vi "DrivePID.vi"(0 "Ldrive Encoder":dbl, 5 "Rdrive Encoder":dbl, 7 "Compensate":bool, 9 "SetpointLeft":dbl format="%.2f", 11 "SetpointRight":dbl format="%.2f") -> (6 "Left Out":dbl, 8 "Right Out":dbl, 15 "Done":bool)   [LabVIEW 2015]
uses:
  <vilib>/addons/control/pid/pid.llb/PID (DBL).vi
  <vilib>/addons/control/pid/NI_PID_pid.lvlib
panel:
  in  "Max Speed":dbl=0.5
  in  "RightDriveRefNum":string="My Encoder RefNum"
  in  "LeftDriveRefNum":string="My Encoder RefNum"
  in  "PID gains for motor gain":T1={"proportional gain (Kc)"=1.0, "integral time (Ti, min)"=0.01, "derivative time (Td, min)"=0.0} {"derivative time (Td, min)" format="%.3f"; "integral time (Ti, min)" format="%.3f"; "proportional gain (Kc)" format="%.3f"}
  in  "PID gains Right":T1={"proportional gain (Kc)"=0.6, "integral time (Ti, min)"=0.0055, "derivative time (Td, min)"=0.001} {"derivative time (Td, min)" format="%.3f"; "integral time (Ti, min)" format="%.7f"; "proportional gain (Kc)" format="%.3f"}
  out "Right Chart":dbl(graph)
  out "Left Chart":dbl(graph)
  in  "PID gains Left":T1={"proportional gain (Kc)"=0.6, "integral time (Ti, min)"=0.0055, "derivative time (Td, min)"=0.001} {"derivative time (Td, min)" format="%.3f"; "integral time (Ti, min)" format="%.7f"; "proportional gain (Kc)" format="%.3f"}
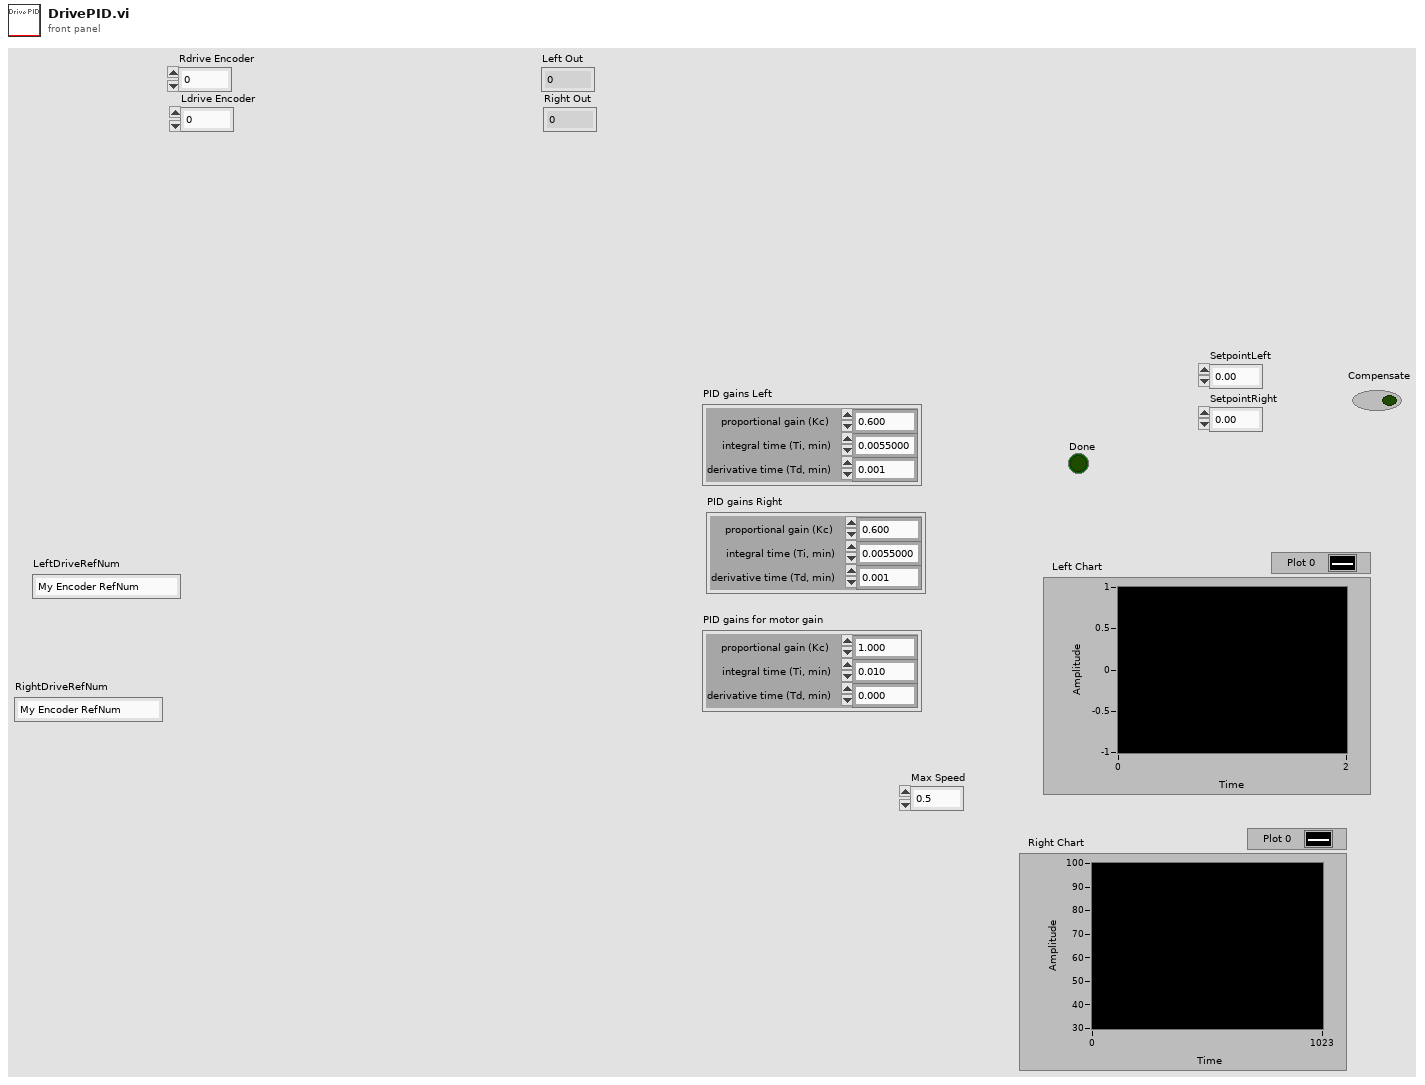
[diagram p1: front panel]
types:
  T1 = cluster{"proportional gain (Kc)":dbl, "integral time (Ti, min)":dbl, "derivative time (Td, min)":dbl}
  T2 = typedef "WPI_EncoderDevRef.ctl" = cluster{"DevStatus":errorcluster, "EncoderIndex":T3, "CounterIndex":T4, "DistancePerCount":dbl, "Decoding Type":T5}
  T3 = typedef "FPGA_EncoderIdx.ctl" = enum8{"Enc 0", "Enc 1", "Enc 2", "Enc 3", "Enc 4", "Enc 5", "Enc 6", "Enc 7", "Invalid"}
  T4 = typedef "FPGA_CounterCtrSystemIndex.ctl" = enum8{"Ctr 0", "Ctr 1", "Ctr 2", "Ctr 3", "Ctr 4", "Ctr 5", "Ctr 6", "Ctr 7", "Invalid"}
  T5 = typedef "WPI_EncoderType.ctl" = enum16{"1x", "2x", "4x"}
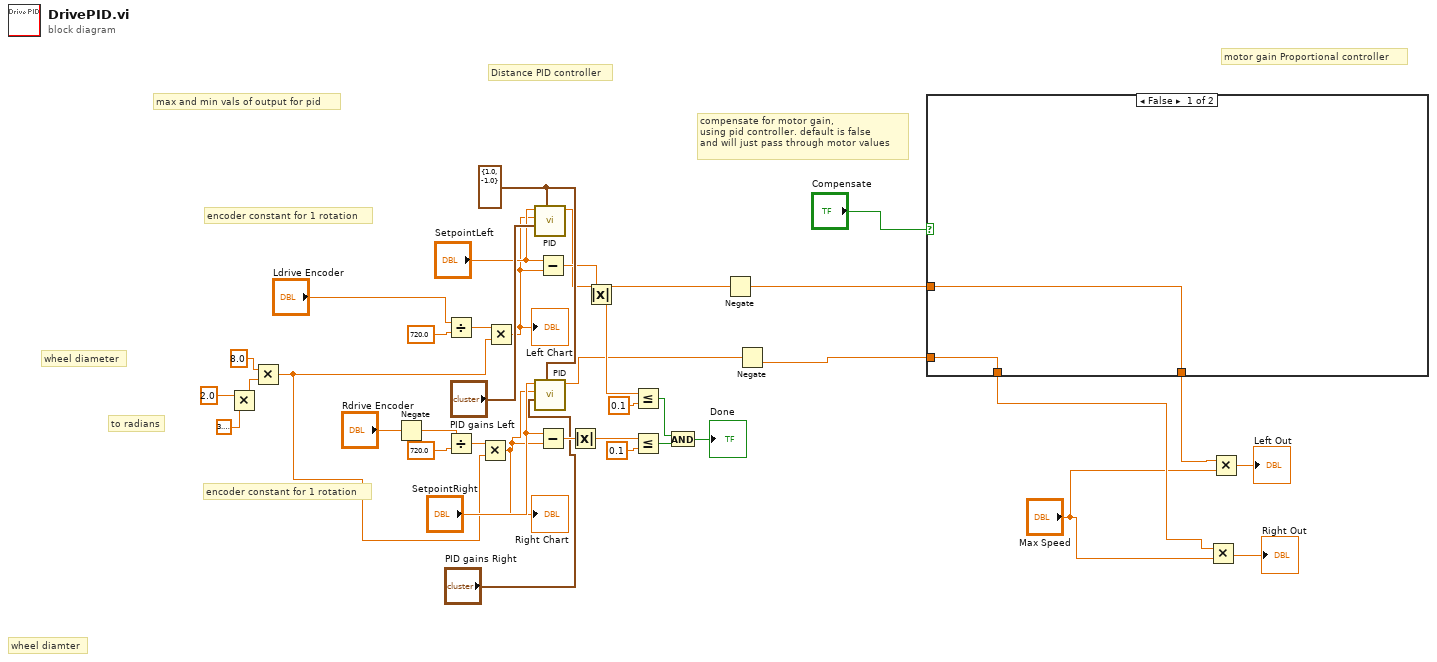
[diagram p0: block diagram]
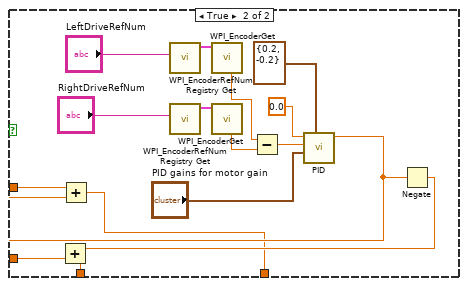
[diagram p2: hidden frame]
diagram:
  w36 = cluster{"output high":dbl, "output low":dbl} {"output high"=1.0, "output low"=-1.0} ("output range")
  # "to radians"
  # "compensate for motor gain,\nusing pid controller. default is false\nand will just pass through motor values"
  # "max and min vals of output for pid"
  # "encoder constant for 1 rotation"
  # "encoder constant for 1 rotation"
  # "wheel diamter"
  # "wheel diameter"
  # "motor gain Proportional controller"
  # "Distance PID controller"
  n1 = Multiply(x=2.0, y=3.141592653589793) -> (x*y=w7:dbl)
  n2 = Multiply(x=8.0, y=w7) -> (x*y=w5:dbl)
  n3 = Negate(x="Rdrive Encoder") -> (-x=w2:dbl)
  n4 = Divide(x="Ldrive Encoder", y=720.0) -> (x/y=w21:dbl)
  n5 = Divide(x=w2, y=720.0) -> (x/y=w19:dbl)
  n6 = Multiply(x=w19, y=w5) -> (x*y=w17:dbl)
  "Right Chart" <- w17
  n7 = Multiply(x=w21, y=w5) -> (x*y=w20:dbl)
  "Left Chart" <- w20
  n8 = call-poly <vilib>:"PID.vi"("output range"=w36, "PID gains"="PID gains Left", "process variable"=w20, "setpoint"="SetpointLeft") -> ("output"=w16:dbl)  [unwired: 6 in, 1 out]
  n9 = call-poly <vilib>:"PID.vi"("output range"=w36, "PID gains"="PID gains Right", "process variable"=w17, "setpoint"="SetpointRight") -> ("output"=w3:dbl)  [unwired: 6 in, 1 out]
  n10 = Subtract(x="SetpointLeft", y=w20) -> (x-y=w34:dbl)
  n11 = Subtract(x="SetpointRight", y=w17) -> (x-y=w28:dbl)
  n12 = Absolute Value(x=w28) -> (abs(x)=w22:dbl)
  n13 = Absolute Value(x=w34) -> (abs(x)=w23:dbl)
  n14 = Less Or Equal?(x=w23, y=0.1) -> (x <= y?=w31:bool)
  n15 = Less Or Equal?(x=w22, y=0.1) -> (x <= y?=w32:bool)
  n16 = And(x=w31, y=w32) -> (x .and. y?=→"Done":bool)
  n17 = Negate(x=w16) -> (-x=w8:dbl)
  n18 = Negate(x=w3) -> (-x=w1:dbl)
  n19 = case shown="False" "Compensate" {
    tunnel: w1 -> [w39 w46]
    tunnel: [w39 w44] -> w13
    tunnel: w8 -> [w40 w43]
    tunnel: [w40 w41] -> w14
    frame False {
    }
    frame True {
      n20 = call <vilib>:"WPI_EncoderRefNum Registry Get.vi"("refnum name"="LeftDriveRefNum") -> ("EncoderDevRef"=w55:T2)  [unwired: 9 in, 1 out]
      n21 = call <vilib>:"WPI_EncoderRefNum Registry Get.vi"("refnum name"="RightDriveRefNum") -> ("EncoderDevRef"=w52:T2)  [unwired: 9 in, 1 out]
      n22 = call <vilib>:"WPI_EncoderGet.vi"("EncoderDevRef"=w55) -> ("Rate"=w50:dbl)  [unwired: 5 in, 5 out]
      n23 = call <vilib>:"WPI_EncoderGet.vi"("EncoderDevRef"=w52) -> ("Rate"=w49:dbl)  [unwired: 5 in, 5 out]
      n24 = Subtract(x=w50, y=w49) -> (x-y=w47:dbl)
      n25 = call-poly <vilib>:"PID.vi"("output range"=cluster{"output high":dbl, "output low":dbl} {"output high"=0.2, "output low"=-0.2}, "PID gains"="PID gains for motor gain", "process variable"=w47, "setpoint"=0.0) -> ("output"=w42:dbl)  [unwired: 6 in, 1 out]
      n26 = Add(x=w43, y=w42) -> (x+y=w41:dbl)
      n27 = Negate(x=w42) -> (-x=w45:dbl)
      n28 = Add(x=w45, y=w46) -> (x+y=w44:dbl)
    }
  }
  n29 = Multiply(x=w13, y="Max Speed") -> (x*y=→"Right Out":dbl)
  n30 = Multiply(x=w14, y="Max Speed") -> (x*y=→"Left Out":dbl)
